vi "Configure IF Bandwith.vi"(8 "error in (no error)":errorcluster, 10 "IF BW [Hz]":dbl, 11 "VNA-CMT S2 S4 in":refnum<class "VNA-CMT S2 S4.lvclass">) -> (0 "error out":errorcluster, 2 "IF BW used [Hz]":dbl, 3 "VNA-CMT S2 S4 out":refnum<class "VNA-CMT S2 S4.lvclass">)   [LabVIEW 2020, in "VNA-CMT S2 S4.lvclass"]
doc: "Configures the Intermidiate Frequency Bandwidth. \nIt chooses the closest supported bandwidth.\nIt returns the used IF BW."
uses:
  VNA-CMT S2 S4.lvclass
  C:/Sandbox/RF Bench/Source Code/WiSpry Test Framework/Instruments/Instrument.lvclass
  C:/Sandbox/RF Bench/Source Code/WiSpry Test Framework/Instruments/Vector Network Analyzer/Vector Network Analyzer.lvclass
  Instrument.lvclass/Instrument.ctl
  Vector Network Analyzer.lvclass/Vector Network Analyzer.ctl
  Instrument.lvclass
  <instrlib>/CMT S2 and S4 VNA/CMT S2 and S4 VNA.lvlib
  Vector Network Analyzer.lvclass
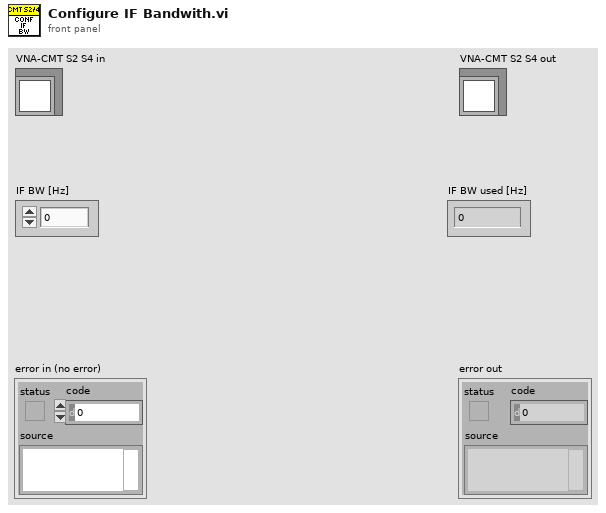
[diagram p1: front panel]
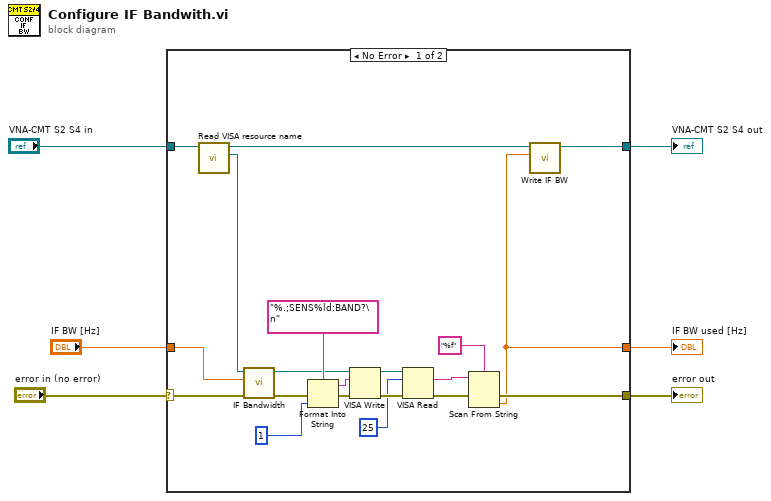
[diagram p0: block diagram]
diagram:
  n1 = case shown="No Error" "error in (no error)" {
    selector: "error in (no error)" -> [w24 w28]
    tunnel: "VNA-CMT S2 S4 in" -> [w26 w29]
    tunnel: [w13 w29] -> w4
    tunnel: [w10 w28] -> w3
    tunnel: "IF BW [Hz]" -> [w23 w27]
    tunnel: [w8 w27] -> w1
    frame No Error {
      n2 = call "Read VISA resource name.vi"("Instrument in"=w26) -> ("VISA resource name"=w25:refnum<visa-resource-name>, "Instrument out"=w14:refnum<class "VNA-CMT S2 S4.lvclass">)  [unwired: 9 in]
      n3 = call <instrlib>:"IF Bandwidth.vi"("error in (no error)"=w24, "IF Bandwidth (10000.0)"=w23, "VISA resource name"=w25) -> ("error out"=w16:errorcluster, "VISA resource name out"=w7:refnum<visa-resource-name>)  [unwired: 7 in]
      n4 = Format Into String(format string="%.;SENS%ld:BAND?\n", error in=w16, 1 ("Channel (1)")) -> (resulting string=w18:string, error out=w17:errorcluster)  [unwired: 1 in]
      n5 = VISA Write(VISA resource name=w7, write buffer=w18, error in (no error)=w17) -> (VISA resource name out=w19:refnum<visa-resource-name>, error out=w20:errorcluster)  [unwired: 1 out]
      n6 = VISA Read(VISA resource name=w19, byte count=u32 25, error in (no error)=w20) -> (read buffer=w12:string, error out=w11:errorcluster)  [unwired: 2 out]
      n7 = Scan From String(format string="%f", input string=w12, error in=w11) -> (error out=w10:errorcluster, output 1=w8:dbl)  [unwired: 2 in, 2 out]
      n8 = call "Write IF BW.vi"("IF BW"=w8, "Vector Network Analyzer in"=w14) -> ("Vector Network Analyzer out"=w13:refnum<class "VNA-CMT S2 S4.lvclass">)  [unwired: 9 in]
    }
    frame Error {
    }
  }
  "error out" <- w3
  "VNA-CMT S2 S4 out" <- w4
  "IF BW used [Hz]" <- w1
